vi "load Test.vi"(8 "error in (no error)":errorcluster caption="Fehler (Eingang, kein Fehler)", 10 "irgendein Test":refnum<class "TestInterface.lvclass">, 11 "DeviceInterface Eingang":refnum<class "DeviceInterface.lvclass"> caption="DNL_LabVIEW Object in") -> (0 "error out":errorcluster caption="Fehler (Ausgang)", 2 "TestInterface.lvclass":refnum<class "TestInterface.lvclass">, 3 "DeviceInterface Ausgang":refnum<class "DeviceInterface.lvclass"> caption="DNL_LabVIEW Object out")   [LabVIEW 2013, in "DeviceInterface.lvclass"]
doc: "Hier kann ein Test ausgewählt werden. Der Nutzer hat die Möglichkeit Tests auszuwählen die als Standardtests hinterlegt sind oder Tests die in den Dateien mit %NORM-NAME%test.json im Programmverzeichznis abgelegt sind. Sollte der Anwender den Dialog abbrechen wird der aktuelle Test durchgeschleift."
uses:
  DeviceInterface.lvclass
  Tests/TestInterface/TestInterface.lvclass
  choosetest.ctl
  choosetestdata.ctl
  Tests/Burst/Burst.lvclass
  Tests/HF-Felder/HF-Felder.lvclass
  Tests/Stoeraussendung/Stoeraussendung.lvclass
  Tests/Surge/Surge.lvclass
  Tests/Spannungseinbruch/Spannungseinbruch.lvclass
  Tests/ESD/ESD.lvclass
  lib/DataCreation.lvlib
panel:
  in  "Cancel Button":bool
  in  "OK Button":bool
  in  "Listenfeld":i32(listbox)
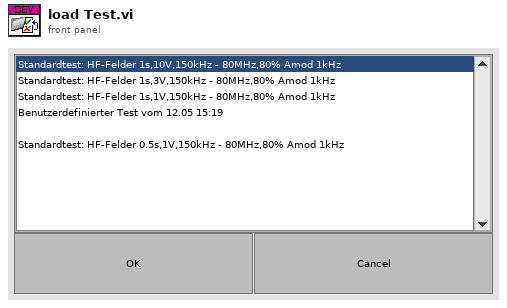
[diagram p1: front panel]
types:
  T1 = typedef "choosetestdata.ctl" = cluster{"number of standard tests":i32, "Path":path}
  T2 = typedef "choosetest.ctl" = enum16{"merge standard with saved Tests", "edit copy of Test", "write Test DB", "event loop", "populate List", "delete Test", "edit Test"}
  T3 = enum16{"open", "replace", "create", "open or create", "replace or create", "replace or create with confirmation"}
  T4 = typedef "eventvkey.ctl" = enum16{"ASCII", "Enter", "Return", "Shift", "Ctrl", "Alt", "Cmd", "Opt", "Caps", "NumLock", "Clear", "Break", "Up", "Down", "Left", "Right", "Insert", "Delete", "Home", "End", "PageUp", "PageDown", "Escape", "Help", "Pause", "ScrollLock", "F1", "F2", "F3", "F4", "F5", "F6", "F7", "F8", "F9", "F10", "F11", "F12", "F13", "F14", "F15", "F16", "F17", "F18", "F19", "F20", "F21", "F22", "F23", "F24", "Play", "VolumeUp", "VolumeDown", "Mute", "Two Byte Char"}
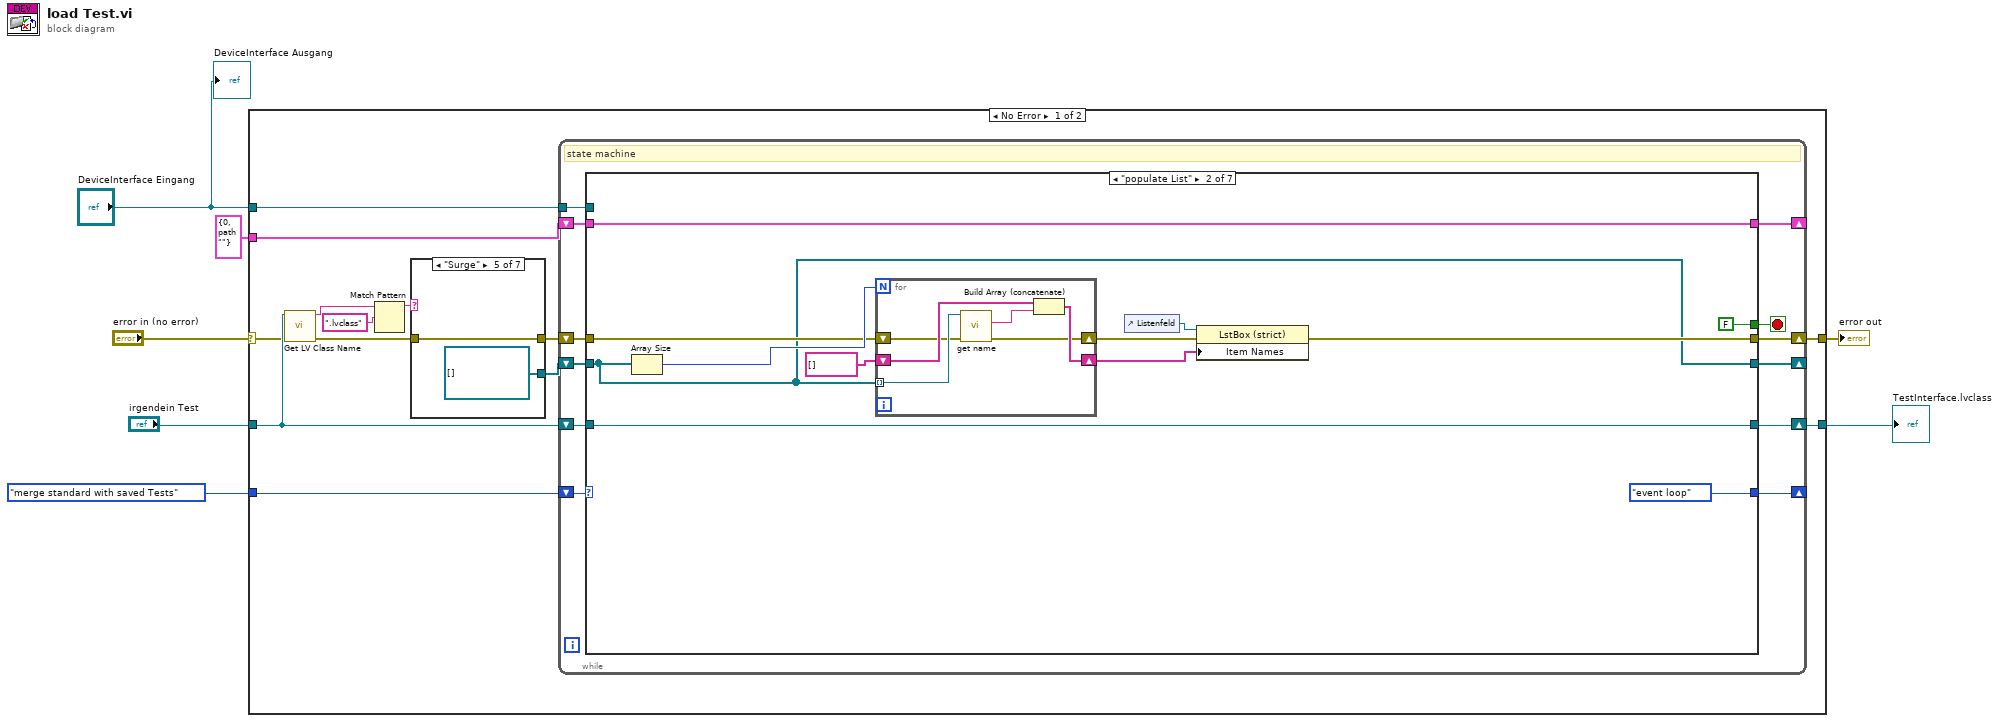
[diagram p0: block diagram]
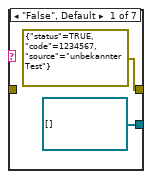
[diagram p2: hidden frame]
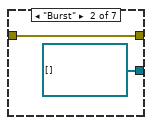
[diagram p3: hidden frame]
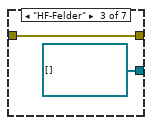
[diagram p4: hidden frame]
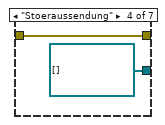
[diagram p5: hidden frame]
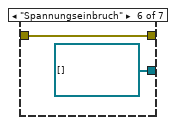
[diagram p6: hidden frame]
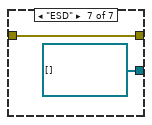
[diagram p7: hidden frame]
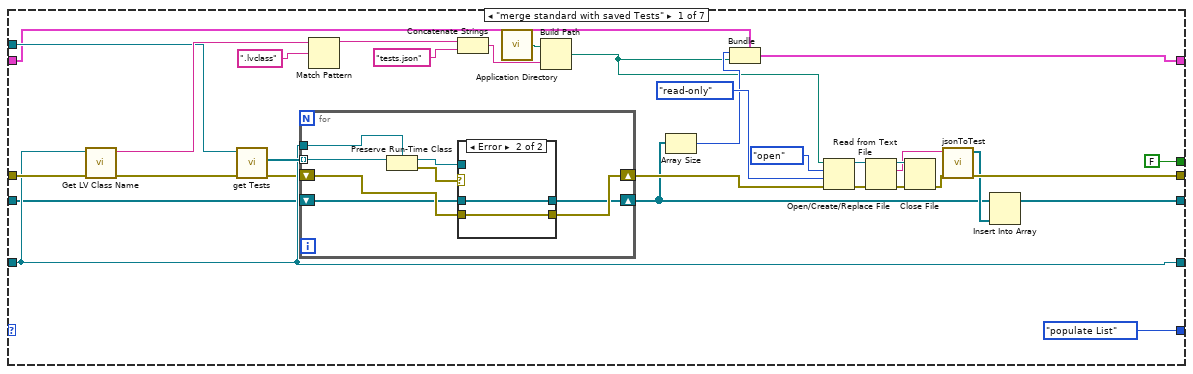
[diagram p8: hidden frame]
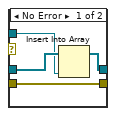
[diagram p9: hidden frame]
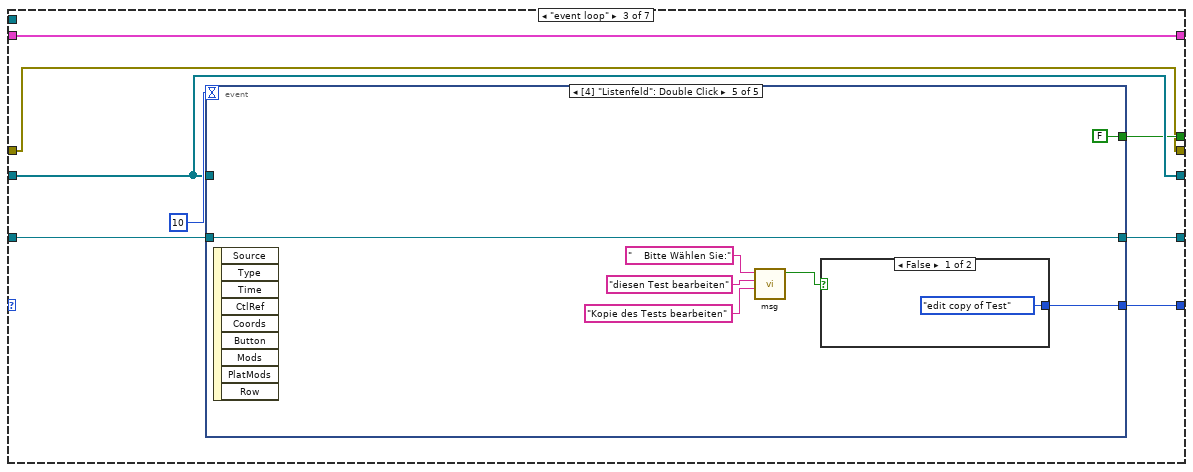
[diagram p10: hidden frame]
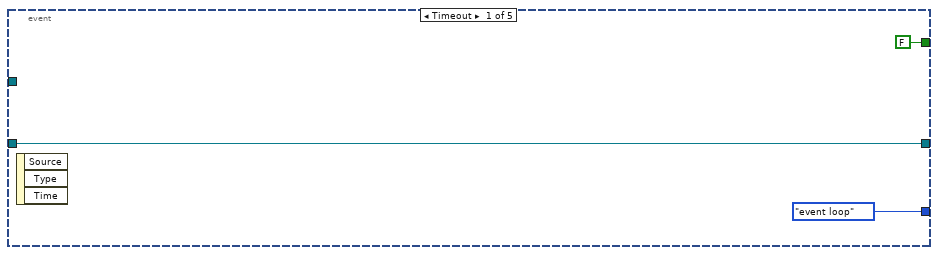
[diagram p11: hidden frame]
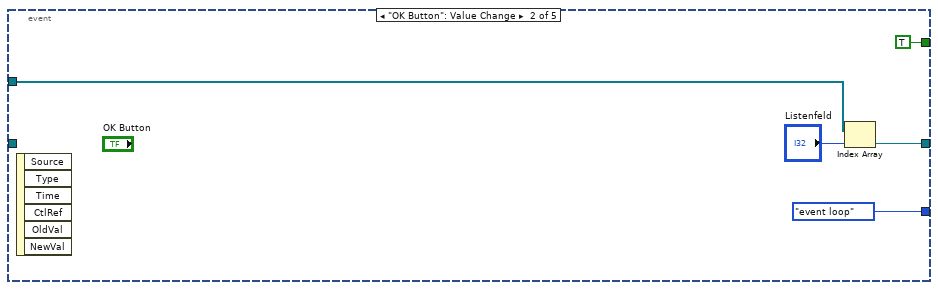
[diagram p12: hidden frame]
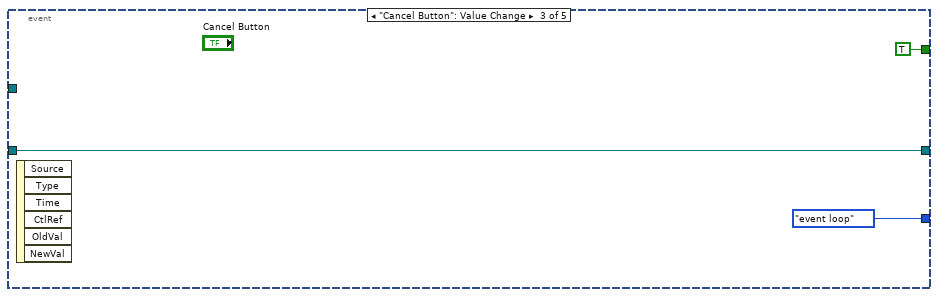
[diagram p13: hidden frame]
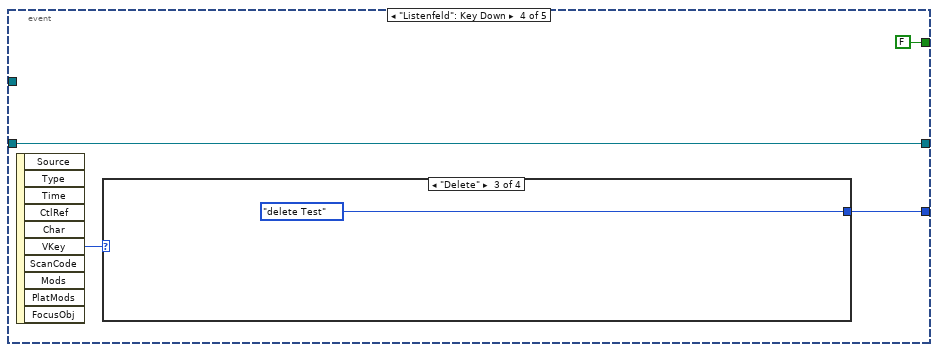
[diagram p14: hidden frame]
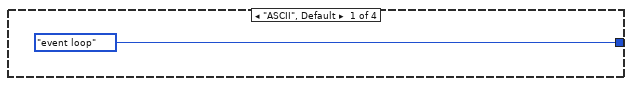
[diagram p15: hidden frame]
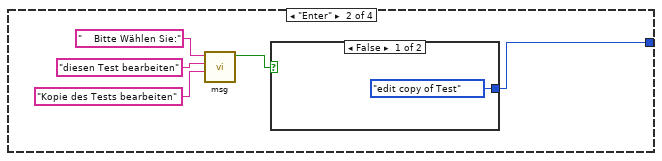
[diagram p16: hidden frame]
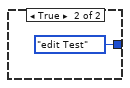
[diagram p17: hidden frame]
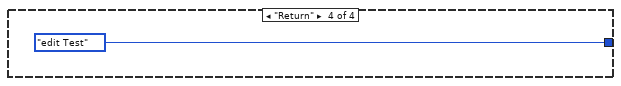
[diagram p18: hidden frame]
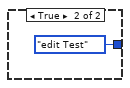
[diagram p19: hidden frame]
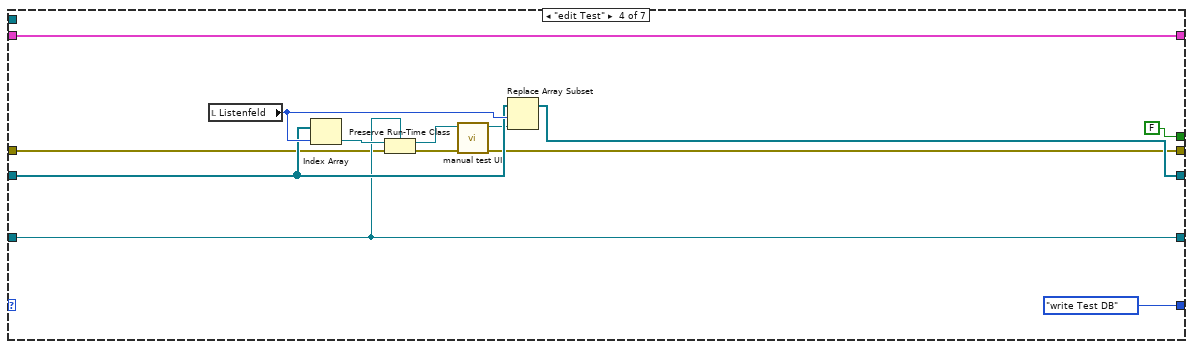
[diagram p20: hidden frame]
diagram:
  n1 = case shown="No Error" "error in (no error)" {
    selector: "error in (no error)" -> [w13 w220]
    tunnel: [w20 w220] -> w6
    tunnel: "irgendein Test" -> [w14 w219]
    tunnel: "DeviceInterface Eingang" -> [w19 _]
    tunnel: choosetest."merge standard with saved Tests" -> [w18 _]
    tunnel: [w16 w219] -> w3
    tunnel: T1 {"number of standard tests"=0, "Path"=path ""} ("Cluster") -> [w15 _]
    frame No Error {
      n2 = call <vilib>:"Get LV Class Name.vi"("error in (no error)"=w13, "object"=w14) -> ("error out"=w9:errorcluster, "class name"=w11:string)  [unwired: 8 in]
      n3 = Match Pattern(string=w11, regular expression=".lvclass") -> (before substring=w10:string)  [unwired: 1 in, 3 out]
      n4 = case shown="\"Surge\"" w10 {
        tunnel: [refnum<class "TestInterface.lvclass">[] [] ("Tests") refnum<class "Burst.lvclass">[] [] ("Tests") refnum<class "HF-Felder.lvclass">[] [] ("Tests") refnum<class "Stoeraussendung.lvclass">[] [] ("Tests") refnum<class "Surge.lvclass">[] [] ("Tests") refnum<class "Spannungseinbruch.lvclass">[] [] ("Tests") refnum<class "ESD.lvclass">[] [] ("Tests")] -> w17
        tunnel: w9 -> [_ w23 w25 w27 w29 w31 w33]
        tunnel: [errorcluster {"status"=TRUE, "code"=1234567, "source"="unbekannter Test"} ("error constant") w23 w25 w27 w29 w31 w33] -> w8
        frame "False", Default {
        }
        frame "Burst" {
        }
        frame "HF-Felder" {
        }
        frame "Stoeraussendung" {
        }
        frame "Surge" {
        }
        frame "Spannungseinbruch" {
        }
        frame "ESD" {
        }
      }
      n5 = while {
        shift-right: [w35] -> w20
        shift-left: w8 -> [w45]
        tunnel: w19 -> [w44]
        shift-right: [w42] -> _
        shift-left: w17 -> [w41]
        shift-right: [w40] -> _
        shift-left: w18 -> [w43]
        shift-right: [w39] -> w16
        shift-left: w14 -> [w46]
        shift-right: [w36] -> _
        shift-left: w15 -> [w37]
        stop <- w38 stop-if-true
        # "state machine"
        n6 = case shown="\"populate List\"" w43 {
          tunnel: w46 -> [w51 w93 w114 w156 w174 w184 w204]
          tunnel: w45 -> [w64 w95 w112 w153 w169 w185 w197]
          tunnel: w44 -> [w62 _ _ _ _ _ _]
          tunnel: [w61 w94 w116 w160 w167 w180 w198] -> w42
          tunnel: w41 -> [w50 w94 w116 w161 w168 w180 w203]
          tunnel: [choosetest."populate List" choosetest."event loop" w117 choosetest."write Test DB" choosetest."write Test DB" choosetest."populate List" choosetest."write Test DB"] -> w40
          tunnel: [w51 w93 w115 w156 w174 w184 w204] -> w39
          tunnel: [FALSE FALSE w113 FALSE FALSE FALSE FALSE] -> w38
          tunnel: w37 -> [w59 w98 w111 w163 w176 w183 w201]
          tunnel: [w58 w98 w111 w163 w176 w183 w201] -> w36
          tunnel: [w55 w96 w112 w159 w175 w182 w197] -> w35
          frame "merge standard with saved Tests" {
            n7 = call <vilib>:"Get LV Class Name.vi"("error in (no error)"=w64, "object"=w51) -> ("error out"=w63:errorcluster, "class name"=w77:string)  [unwired: 8 in]
            n8 = call-dynamic "get Tests.vi"("error in (no error)"=w63, "DeviceInterface (Eingang)"=w62) -> ("error out"=w49:errorcluster, "Tests"=w52:refnum<class "TestInterface.lvclass">[])  [unwired: 7 in, 1 out]
            n9 = for {
              tunnel: w52 -> [w85] mode=indexing
              shift-right: [w86] -> w48
              shift-left: w49 -> [w83]
              tunnel: w51 -> [w82]
              shift-right: [w79] -> w47
              shift-left: w50 -> [w81]
              n10 = Preserve Run-Time Class(object in=w85, 2:w82) -> (object out=w80:refnum<class "TestInterface.lvclass">, error out=w84:errorcluster)  [unwired: 1 in]
              n11 = case shown="Error" w84 {
                tunnel: w83 -> [w90 w92]
                tunnel: [w90 w92] -> w86
                tunnel: w81 -> [w89 w91]
                tunnel: w80 -> [w88 _]
                tunnel: [w87 w91] -> w79
                frame No Error {
                  n12 = Insert Into Array(array=w89, new element=w88) -> (w87:refnum<class "TestInterface.lvclass">[])  [unwired: 1 in]
                }
                frame Error {
                }
              }
            }
            n13 = Match Pattern(string=w77, regular expression=".lvclass") -> (before substring=w78:string)  [unwired: 1 in, 3 out]
            n14 = Concatenate Strings(w78, "tests.json" ("string")) -> (w74:string)
            n15 = call <vilib>:"Application Directory.vi"() -> ("Application Directory"=w75:path)
            n16 = Build Path(base path=w75, name or relative path=w74) -> (appended path=w54:path)
            n17 = Array Size(array=w47) -> (size(s)=w60:i32)
            n18 = Bundle(cluster=w59, "number of standard tests"=w60, "Path"=w54) -> (w58:T1)
            n19 = Open/Create/Replace File(file path (use dialog)=w54, error in=w48, operation (0:open)=T3."open", access (0:read/write)=enum16{"read/write", "read-only", "write-only"}."read-only") -> (refnum out=w70:refnum<file>, error out=w69:errorcluster)  [unwired: 2 in, 1 out]
            n20 = Read from Text File(file (use dialog)=w70, error in=w69) -> (refnum out=w67:refnum<file>, text=w66:string, error out=w68:errorcluster)  [unwired: 2 in, 1 out]
            n21 = Close File(refnum=w67, error in=w68) -> (error out=w65:errorcluster)  [unwired: 1 out]
            n22 = call "jsonToTest.vi"("error in (no error)"=w65, "JSON string"=w66) -> ("error out"=w55:errorcluster, "Tests"=w53:refnum<class "TestInterface.lvclass">[])  [unwired: 8 in]
            n23 = Insert Into Array(array=w47, new element=w53) -> (w61:refnum<class "TestInterface.lvclass">[])  [unwired: 1 in]
          }
          frame "populate List" {
            n24 = Array Size(array=w94) -> (size(s)=w103:i32)
            n25 = for {
              N: w103 -> [_]
              tunnel: w94 -> [w107] mode=indexing
              shift-right: [w110] -> w100
              shift-left: string[] [] -> [w109]
              shift-right: [w108] -> w101
              shift-left: w95 -> [w106]
              n26 = call-dynamic "get name.vi"("error in (no error)"=w106, "TestInterface (Eingang)"=w107) -> ("error out"=w108:errorcluster, "name"=w105:string)  [unwired: 7 in, 1 out]
              n27 = Build Array (concatenate)(w109, w105) -> (w110:string[])
            }
            n28 = control-ref of="Listenfeld"() -> (w102:refnum<vi>)
            n29 = property class="LstBox (strict)"(reference=w102, error in=w101, "Item Names"=w100) -> (error out=w96:errorcluster)  [unwired: 1 out]
          }
          frame "event loop" {
            n30 = event shown="[4] \"Listenfeld\": Double Click" {
              selector: _ -> [_ _ _ _ _]
              dyn-events: _ -> [_ _ _ _ _]
              timeout: 10 -> [_ _ _ _ _]
              tunnel: [choosetest."event loop" choosetest."event loop" choosetest."event loop" w132 w149] -> w117
              tunnel: w116 -> [_ w126 _ _ _]
              tunnel: [w120 w124 w129 w130 w148] -> w115
              tunnel: w114 -> [w120 _ w129 w130 w148]
              tunnel: [FALSE TRUE TRUE FALSE FALSE] -> w113
              event Timeout {
                n31 = event-data() -> ()  [unwired: 1 in, 3 out]
              }
              event "OK Button": Value Change {
                n32 = event-data() -> ()  [unwired: 1 in, 6 out]
                n33 = Index Array(array=w126, index="Listenfeld") -> (element=w124:refnum<class "TestInterface.lvclass">)
              }
              event "Cancel Button": Value Change {
                n34 = event-data() -> ()  [unwired: 1 in, 6 out]
              }
              event "Listenfeld": Key Down {
                n35 = event-data() -> ("VKey"=w133:T4)  [unwired: 1 in, 9 out]
                n36 = case shown="\"Delete\"" w133 {
                  tunnel: [choosetest."event loop" w135 choosetest."delete Test" choosetest."edit Test"] -> w132
                  frame "ASCII", Default {
                  }
                  frame "Enter" {
                    n37 = call "msg.vi"("F button name (\"Cancel\")"="Kopie des Tests bearbeiten" ("F button name (\"Cancel\")"), "T button name (\"OK\")"="diesen Test bearbeiten" ("T button name (\"OK\")"), "message"="    Bitte Wählen Sie:") -> ("T button?"=w136:bool)  [unwired: 8 in]
                    n38 = case shown="False" w136 {
                      tunnel: [choosetest."edit copy of Test" choosetest."edit Test"] -> w135
                      frame False {
                      }
                      frame True {
                      }
                    }
                  }
                  frame "Delete" {
                  }
                  frame "Return" {
                  }
                }
              }
              event "Listenfeld": Double Click {
                n39 = event-data() -> ()  [unwired: 1 in, 9 out]
                n40 = call "msg.vi"("F button name (\"Cancel\")"="Kopie des Tests bearbeiten" ("F button name (\"Cancel\")"), "T button name (\"OK\")"="diesen Test bearbeiten" ("T button name (\"OK\")"), "message"="    Bitte Wählen Sie:") -> ("T button?"=w144:bool)  [unwired: 8 in]
                n41 = case shown="False" w144 {
                  tunnel: [choosetest."edit copy of Test" choosetest."edit Test"] -> w149
                  frame False {
                  }
                  frame True {
                  }
                }
              }
            }
          }
          frame "edit Test" {
            n42 = local read "Listenfeld"() -> (w162:i32)
            n43 = Index Array(array=w161, index=w162) -> (element=w157:refnum<class "TestInterface.lvclass">)
            n44 = Preserve Run-Time Class(object in=w157, error in=w153, 2:w156) -> (object out=w155:refnum<class "TestInterface.lvclass">, error out=w154:errorcluster)
            n45 = call-dynamic "manual test UI.vi"("error in (no error)"=w154, "TestInterface Eingang"=w155) -> ("error out"=w159:errorcluster, "TestInterface Ausgang"=w158:refnum<class "TestInterface.lvclass">)  [unwired: 6 in, 2 out]
            n46 = Replace Array Subset(array=w161, new element=w158, index=w162) -> (w160:refnum<class "TestInterface.lvclass">[])
          }
          frame "edit copy of Test" {
            n47 = local read "Listenfeld"() -> (w170:i32)
            n48 = Index Array(array=w168, index=w170) -> (element=w173:refnum<class "TestInterface.lvclass">)
            n49 = Preserve Run-Time Class(object in=w173, error in=w169, 2:w174) -> (object out=w172:refnum<class "TestInterface.lvclass">, error out=w171:errorcluster)
            n50 = call-dynamic "manual test UI.vi"("error in (no error)"=w171, "TestInterface Eingang"=w172) -> ("error out"=w175:errorcluster, "TestInterface Ausgang"=w166:refnum<class "TestInterface.lvclass">)  [unwired: 6 in, 2 out]
            n51 = Insert Into Array(array=w168, new element=w166) -> (w167:refnum<class "TestInterface.lvclass">[])  [unwired: 1 in]
          }
          frame "write Test DB" {
            n52 = Unbundle By Name(w183) -> ("number of standard tests"=w181:i32, "Path"=w186:path)
            n53 = Array Subset(array=w180, index=w181) -> (w179:refnum<class "TestInterface.lvclass">[])  [unwired: 1 in]
            n54 = call "TestsToJson.vi"("error in (no error)"=w185, "Test Array"=w179) -> ("error out"=w192:errorcluster, "JSON string"=w193:string)  [unwired: 8 in]
            n55 = Open/Create/Replace File(file path (use dialog)=w186, error in=w192, operation (0:open)=T3."replace or create", access (0:read/write)=enum16{"read/write", "read-only", "write-only"}."write-only") -> (refnum out=w194:refnum<file>, error out=w191:errorcluster)  [unwired: 2 in, 1 out]
            n56 = Write to Text File(file (use dialog)=w194, text=w193, error in=w191) -> (refnum out=w189:refnum<file>, error out=w190:errorcluster)  [unwired: 1 in, 1 out]
            n57 = Close File(refnum=w189, error in=w190) -> (error out=w182:errorcluster)  [unwired: 1 out]
          }
          frame "delete Test" {
            n58 = Unbundle(w201) -> ("number of standard tests"=w202:i32)  [unwired: 1 out]
            n59 = local read "Listenfeld"() -> (w199:i32)
            n60 = Greater Or Equal?(x=w199, y=w202) -> (x >= y?=w200:bool)
            n61 = case shown="False" w200 {
              tunnel: w203 -> [w209 w214]
              tunnel: w199 -> [_ w213]
              tunnel: [w209 w212] -> w198
              frame False {
                n62 = One Button Dialog(message="Standardtests können nicht gelöscht werden", button name ("OK")="Ok") -> ()  [unwired: 1 out]
              }
              frame True {
                n63 = Two Button Dialog(message="Soll der Test wirklich gelöscht werden ?") -> (T button?=w210:bool)  [unwired: 2 in]
                n64 = case shown="True" w210 {
                  tunnel: w214 -> [w215 w218]
                  tunnel: w213 -> [_ w217]
                  tunnel: [w215 w216] -> w212
                  frame False {
                  }
                  frame True {
                    n65 = Delete From Array(array=w218, index=w217) -> (array with subset deleted=w216:refnum<class "TestInterface.lvclass">[])  [unwired: 1 in, 1 out]
                  }
                }
              }
            }
          }
        }
      }
    }
    frame Error {
    }
  }
  "error out" <- w6
  "TestInterface.lvclass" <- w3
  "DeviceInterface Ausgang" <- "DeviceInterface Eingang"
